vi "extractDCAOn.vi"(8 "error in (no error)":errorcluster, 11 "ILC in":refnum<class "ILC.lvclass">) -> (0 "error out":errorcluster, 3 "ILC out":refnum<class "ILC.lvclass">)   [LabVIEW 2015, in "ILCCommon.lvlib" / "ILC.lvclass"]
uses:
  <userlib>/Common/ILC/ILC/ILC.lvclass
  <userlib>/Common/ILC/ILC/ILC.lvclass/ILC.ctl
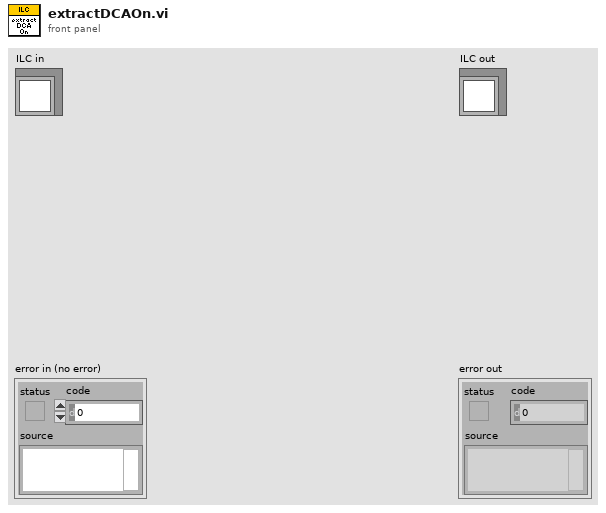
[diagram p1: front panel]
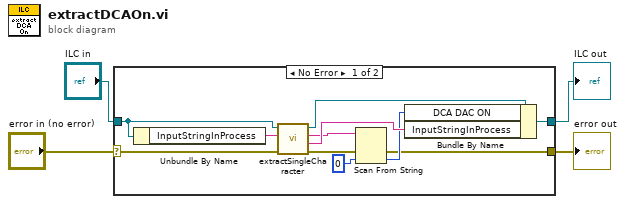
[diagram p0: block diagram]
diagram:
  n1 = case shown="No Error" "error in (no error)" {
    selector: "error in (no error)" -> [w6 w17]
    tunnel: [w5 w17] -> w3
    tunnel: [w12 w16] -> w1
    tunnel: "ILC in" -> [w14 w16]
    frame No Error {
      n2 = Unbundle By Name(w14) -> ("InputStringInProcess"=w15:string)
      n3 = call <userlib>:"extractSingleCharacter.vi"("error in (no error)"=w6, "inputString"=w15, "ILC in"=w14) -> ("error out"=w7:errorcluster, "remainingString"=w11:string, "extractedSegment"=w10:string, "ILC out"=w13:refnum<class "ILC.lvclass">)  [unwired: 5 in]
      n4 = Scan From String(input string=w10, error in=w7, default 1=u16 0) -> (error out=w5:errorcluster, output 1=w8:u16)  [unwired: 2 in, 2 out]
      n5 = Bundle By Name(cluster=w13, "DCA DAC ON"=w8, "InputStringInProcess"=w11) -> (w12:refnum<class "ILC.lvclass">)
    }
    frame Error {
    }
  }
  "error out" <- w3
  "ILC out" <- w1
